vi "String to Binary.vi"() -> ()   [LabVIEW 2015]
panel:
  in  "file path (dialog if empty)":path
  out "Binary String 2":string
  out "unsigned byte array from file":u8[](array[numeric]) format="%.0b"
  out "unsigned byte array":u8[](array[numeric]) format="%.0b"
  out "Binary String 1":string
  in  "String":string="test"
  # "In binary format"
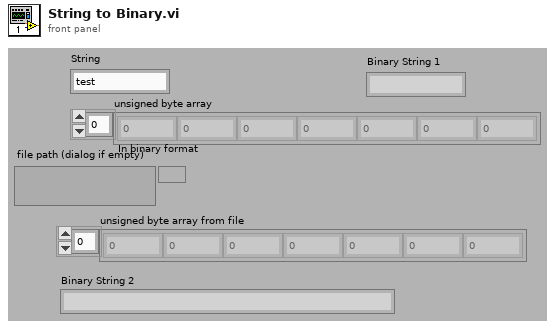
[diagram p1: front panel]
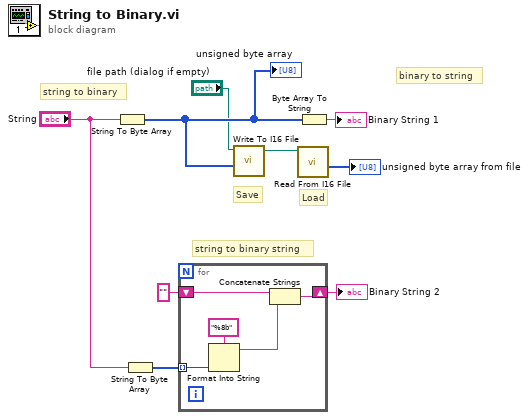
[diagram p0: block diagram]
diagram:
  # "string to binary string"
  # "Load"
  # "Save"
  # "binary to string"
  # "string to binary"
  n1 = String To Byte Array(string="String") -> (unsigned byte array=w8:u8[])
  "unsigned byte array" <- w8
  n2 = String To Byte Array(string="String") -> (unsigned byte array=w4:u8[])
  n3 = for {
    tunnel: w4 -> [w14] mode=indexing
    shift-right: [w12] -> w2
    shift-left: "" -> [w10]
    n4 = Format Into String(format string="%8b" ("Format String"), w14) -> (resulting string=w11:string)  [unwired: 2 in, 1 out]
    n5 = Concatenate Strings(w10, w11) -> (w12:string)
  }
  "Binary String 2" <- w2
  n6 = call <vilib>:"Write To I16 File.vi"("1D array"=w8, "file path (dialog if empty)"="file path (dialog if empty)") -> ("new file path (Not A Path if cancelled)"=w7:path)  [unwired: 5 in]
  n7 = call <vilib>:"Read From I16 File.vi"("file path (dialog if empty)"=w7) -> ("1D array"=→"unsigned byte array from file":i16[])  [unwired: 6 in, 4 out]
  n8 = Byte Array To String(unsigned byte array=w8) -> (string=→"Binary String 1":string)
